vi "B-Spline Fit_nD.vi"(0 "Y":dbl[][](array[numeric]), 1 "# of control points":i32=10, 9 "Weight":dbl[](array[numeric]), 11 "Parameter":dbl[](array[numeric]), 12 "degree":i32=3, 13 "parameter selection":u16(ring)=2 items=["equally spaced", "chord length", "centripetal method"]) -> (4 "BSpline fit Y":dbl[][](array[numeric]), 10 "Control points":dbl[][](array[numeric]), 14 "residue":dbl, 15 "error":i32)   [LabVIEW 2017, in "NI_AALPro.lvlib"]
uses:
  <vilib>/Analysis/NI_AALPro.lvlib
  <resource>/lvanlys.dll
panel:
  # "BSpline Fit (nD)"
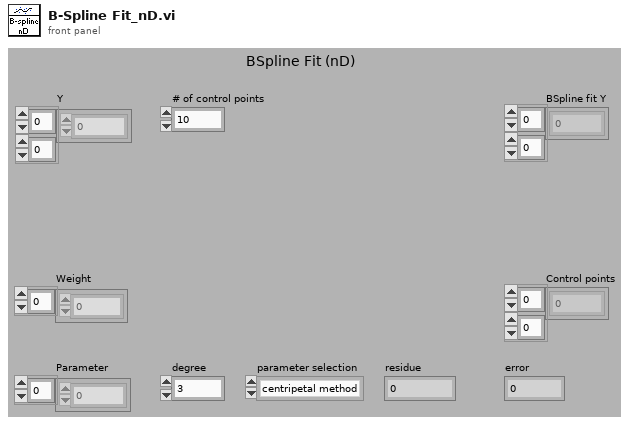
[diagram p1: front panel]
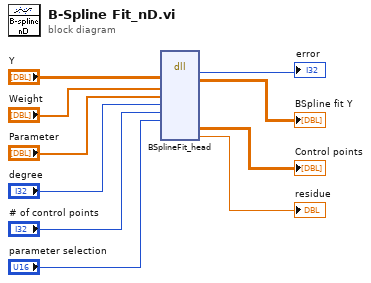
[diagram p0: block diagram]
diagram:
  n1 = dll-call lib="e:/builds/penguin/labview/branches/2017/dev/dist/resource/lvanlys.*" fn="BSplineFit_head"("y"="Y", "weight"="Weight", "parameter"="Parameter", "degree"="degree", "numofCP"="# of control points", "method"="parameter selection") -> ("return type"=→"error":i32, "y"=→"BSpline fit Y":dbl[][], "control points"=→"Control points":dbl[][], "mse"=→"residue":dbl)  [unwired: 8 in, 4 out]
